vi "Arduino_Check_Main_Osciloscope.vi"() -> ()   [LabVIEW 2021]
uses:
  Drivers/Arduino_Pulse_Generator/Configurate/Channel_Pulse_Stream.ctl
  Drivers/Arduino_Pulse_Generator/Configurate/Register_1.ctl
  Drivers/Arduino_Pulse_Generator/Configurate/Register_2.ctl
  <vilib>/Analysis/NI_AALBase.lvlib
panel:
  out "Slide":dbl(slide) scale=0.0..100.0
  out "Histogram Graph":T1(graph)
  out "number of points":i32
  out "alpha unc":dbl format="%0.5f"
  out "alpha":dbl format="%0.2f"
  out "read buffer":string
  out "register 2 (8-13)":T2
  out "register 1 (2-7)":T3
  out "Pulse sequence":T4[](array[typedef]) {"channel" min=2 max=13 step=1}
  out "error out":errorcluster
  in  "error in":errorcluster
  in  "VISA arduino in":refnum<visa-resource-name>
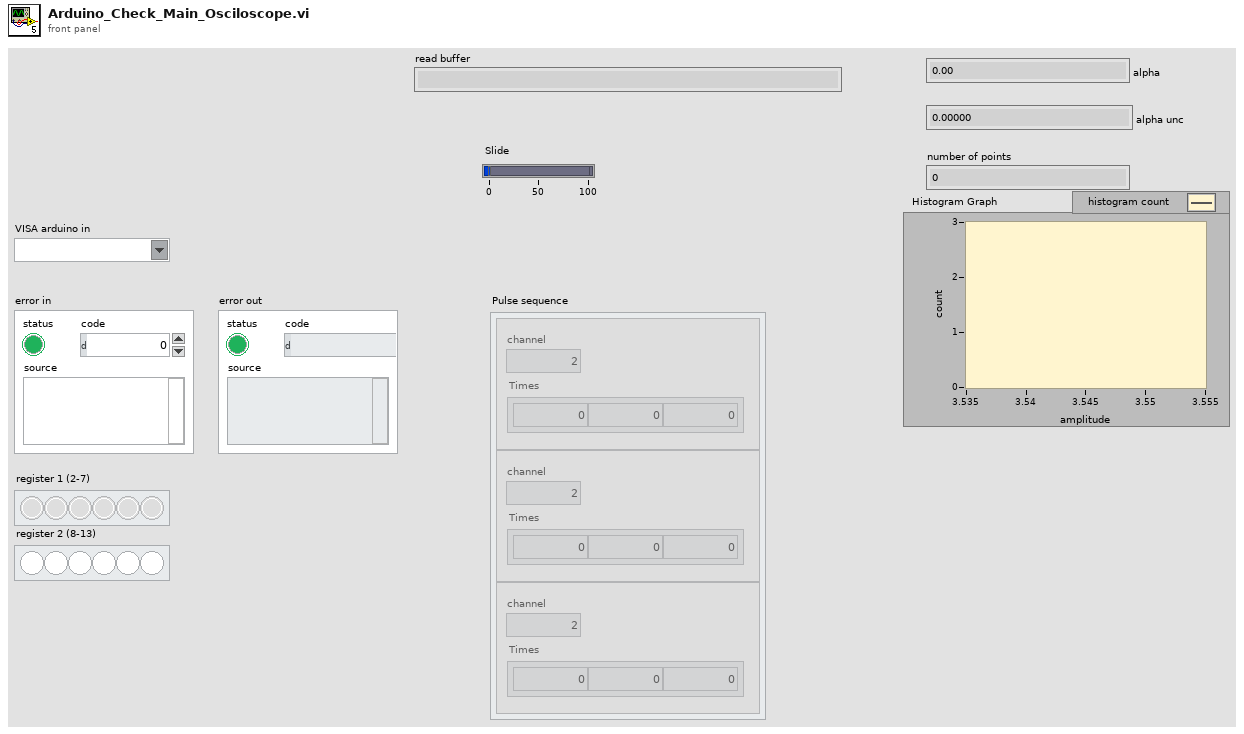
[diagram p1: front panel]
types:
  T1 = cluster{"X Values":dbl[], "Histogram: h(x)":i32[]}
  T2 = typedef "Register_2.ctl" = bool[]
  T3 = typedef "Register_1.ctl" = bool[]
  T4 = typedef "Channel_Pulse_Stream.ctl" = cluster{"Times":dbl[], "channel":u8}
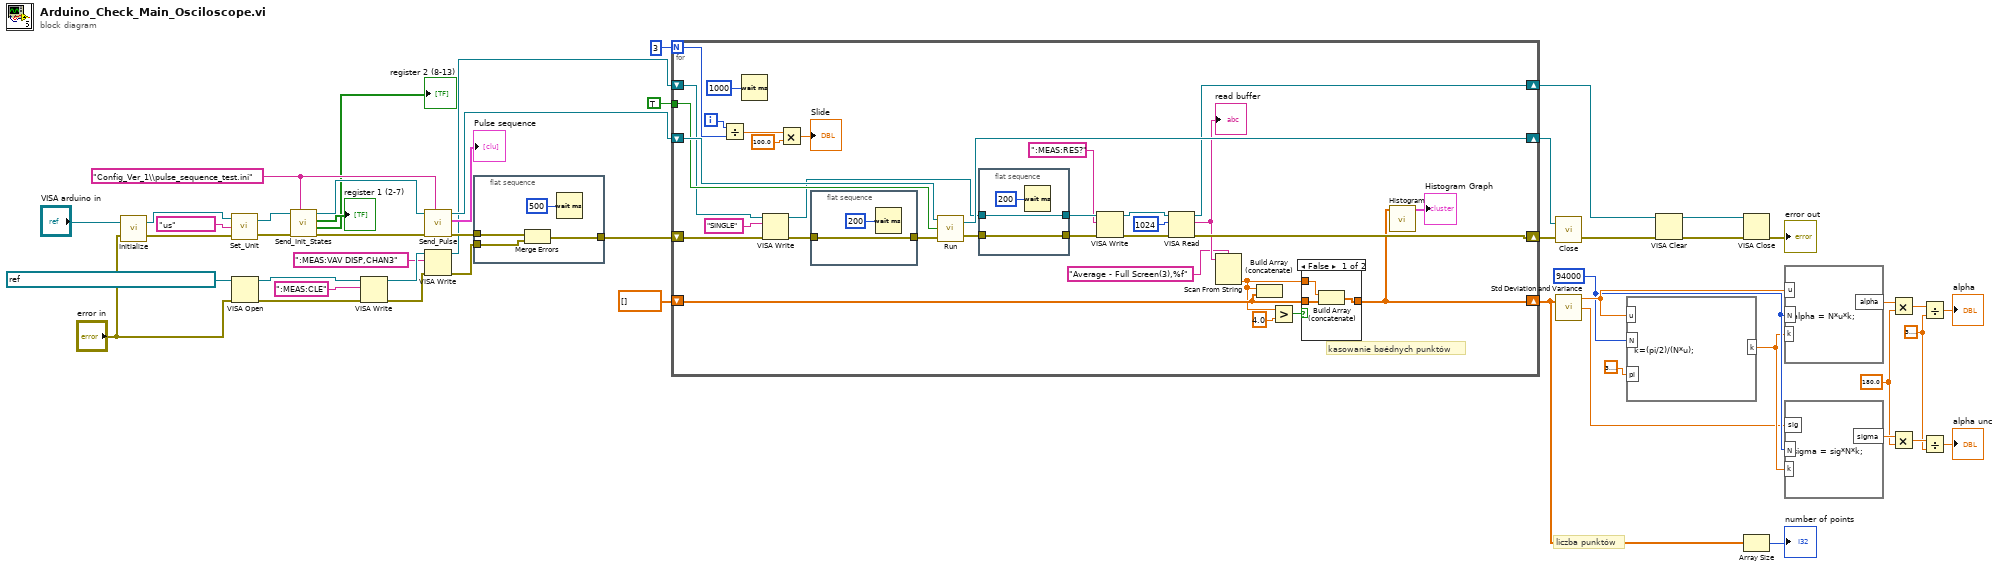
[diagram p0: block diagram]
diagram:
  w5 = 3.141592653589793
  w7 = 180.0 ("y")
  w14 = 94000
  w47 = "Config_Ver_1\\pulse_sequence_test.ini" ("Filename (.ini)")
  # "liczba punktów"
  n1 = call "Initialize.vi"("error in"="error in", "VISA arduino in"="VISA arduino in") -> ("error out"=w42:errorcluster, "VISA arduino out"=w41:refnum<visa-resource-name>)
  n2 = call "Set_Unit.vi"("error in"=w42, "Unit"="us", "VISA arduino in"=w41) -> ("error out"=w44:errorcluster, "VISA arduino out"=w45:refnum<visa-resource-name>)
  n3 = VISA Open(error in (no error)="error in", VISA resource name=refnum<visa-resource-name> "USB0::0x0957::0x1798::MY53280148::INSTR") -> (VISA resource name=w29:refnum<visa-resource-name>, error out=w28:errorcluster)  [unwired: 3 in]
  n4 = call "Send_Init_States.vi"("Filename (.ini)"=w47, "error in"=w44, "VISA arduino in"=w45) -> ("error out"=w48:errorcluster, "register 2 (8-13)"=→"register 2 (8-13)":T2, "register 1 (2-7)"=→"register 1 (2-7)":T3, "VISA arduino out"=w49:refnum<visa-resource-name>)  [unwired: 5 in]
  n5 = VISA Write(VISA resource name=w29, write buffer=":MEAS:CLE", error in (no error)=w28) -> (VISA resource name out=w26:refnum<visa-resource-name>, error out=w25:errorcluster)  [unwired: 1 out]
  n6 = call "Send_Pulse.vi"("Filename (.ini)"=w47, "error in"=w48, "VISA arduino in"=w49) -> ("error out"=w34:errorcluster, "Pulse sequence"=→"Pulse sequence":T4[], "VISA arduino out"=w46:refnum<visa-resource-name>)  [unwired: 6 in]
  n7 = VISA Write(VISA resource name=w26, write buffer=":MEAS:VAV DISP,CHAN3", error in (no error)=w25) -> (VISA resource name out=w22:refnum<visa-resource-name>, error out=w23:errorcluster)  [unwired: 1 out]
  n8 = flat-sequence {
    tunnel: [w51] -> w35
    tunnel: w34 -> [w53]
    tunnel: w23 -> [w52]
    frame #0 {
      n9 = Merge Errors(w53, w52) -> (w51:errorcluster)
      n10 = Wait (ms)(milliseconds to wait=u32 500) -> ()  [unwired: 1 out]
    }
  }
  n11 = for {
    N: 3 -> [w55]
    tunnel: TRUE ("run?") -> [w85]
    shift-right: [w84] -> w39
    shift-left: w46 -> [w86]
    shift-right: [w71] -> w33
    shift-left: w35 -> [w83]
    shift-right: [w72] -> w21
    shift-left: w22 -> [w81]
    shift-right: [w60] -> w1
    shift-left: dbl[] [] -> [w63]
    i -> [w56]
    # "kasowanie bøédnych punktów"
    n12 = Divide(x=w56, y=w55) -> (x/y=w58:dbl)
    n13 = Wait (ms)(milliseconds to wait=u32 1000) -> ()  [unwired: 1 out]
    n14 = VISA Write(VISA resource name=w81, write buffer="SINGLE", error in (no error)=w83) -> (VISA resource name out=w78:refnum<visa-resource-name>, error out=w69:errorcluster)  [unwired: 1 out]
    n15 = Multiply(x=w58, y=100.0) -> (x*y=→"Slide":dbl)
    n16 = flat-sequence {
      tunnel: w69 -> [w91]
      tunnel: [w91] -> w68
      frame #0 {
        n17 = Wait (ms)(milliseconds to wait=u32 200) -> ()  [unwired: 1 out]
      }
    }
    n18 = call "Run.vi"("error in"=w68, "run?"=w85, "VISA arduino in"=w86) -> ("error out"=w80:errorcluster, "VISA arduino out"=w84:refnum<visa-resource-name>)
    n19 = flat-sequence {
      tunnel: w80 -> [w94]
      tunnel: [w94] -> w79
      tunnel: w78 -> [w93]
      tunnel: [w93] -> w77
      frame #0 {
        n20 = Wait (ms)(milliseconds to wait=u32 200) -> ()  [unwired: 1 out]
      }
    }
    n21 = VISA Write(VISA resource name=w77, write buffer=":MEAS:RES?", error in (no error)=w79) -> (VISA resource name out=w75:refnum<visa-resource-name>, error out=w74:errorcluster)  [unwired: 1 out]
    n22 = VISA Read(VISA resource name=w75, byte count=u32 1024, error in (no error)=w74) -> (VISA resource name out=w72:refnum<visa-resource-name>, read buffer=w67:string, error out=w71:errorcluster)  [unwired: 1 out]
    "read buffer" <- w67
    n23 = Scan From String(format string="Average - Full Screen(3),%f", input string=w67) -> (output 1=w62:dbl)  [unwired: 3 in, 3 out]
    n24 = Build Array (concatenate)(w62, w63) -> ()  [unwired: 1 out]
    n25 = Greater?(x=w62, y=4.0) -> (0:w65:bool)
    n26 = case shown="False" w65 {
      tunnel: [w87 w90] -> w60
      tunnel: w63 -> [w88 w90]
      tunnel: w62 -> [w89 _]
      frame False {
        n27 = Build Array (concatenate)(w89, w88) -> (w87:dbl[])
      }
      frame True {
      }
    }
    n28 = call <vilib>:"Histogram.vi"("X"=w60) -> ("Histogram Graph"=→"Histogram Graph":T1)  [unwired: 7 in, 3 out]
  }
  n29 = call "Close.vi"("error in"=w33, "VISA arduino in"=w39) -> ("error out"=w20:errorcluster)  [unwired: 1 in]
  n30 = call <vilib>:"Std Deviation and Variance.vi"("X"=w1) -> ("mean"=w15:dbl, "standard deviation"=w12:dbl)  [unwired: 1 in, 1 out]
  n31 = formula code="k=(pi/2)/(N*u);"("N"=w14, "u"=w15, "pi"=3.141592653589793) -> ("k"=w13:dbl)
  n32 = VISA Clear(VISA resource name=w21, error in (no error)=w20) -> (VISA resource name out=w18:refnum<visa-resource-name>, error out=w19:errorcluster)
  n33 = VISA Close(VISA resource name=w18, error in (no error)=w19) -> (error out=→"error out":errorcluster)
  n34 = Array Size(array=w1) -> (size(s)=→"number of points":i32)
  n35 = formula code="alpha = N*u*k;"("k"=w13, "N"=w14, "u"=w15) -> ("alpha"=w9:dbl)
  n36 = formula code="sigma = sig*N*k;"("k"=w13, "N"=w14, "sig"=w12) -> ("sigma"=w10:dbl)
  n37 = Multiply(x=w9, y=w7) -> (x*y=w8:dbl)
  n38 = Multiply(x=w10, y=w7) -> (x*y=w6:dbl)
  n39 = Divide(x=w8, y=w5) -> (x/y=→"alpha":dbl)
  n40 = Divide(x=w6, y=w5) -> (x/y=→"alpha unc":dbl)
